vi "get_all_sensor_thicknesses.vi"(8 "error in (no error)":errorcluster, 11 "VISA resource name":refnum<visa-resource-name>) -> (0 "error out":errorcluster, 2 "Thickness array (kA)":dbl[](array[numeric]), 3 "VISA resource name out":refnum<visa-resource-name>)   [LabVIEW 2018]
doc: "Query all sendor thicknesses. Returns thicknesses in kA."
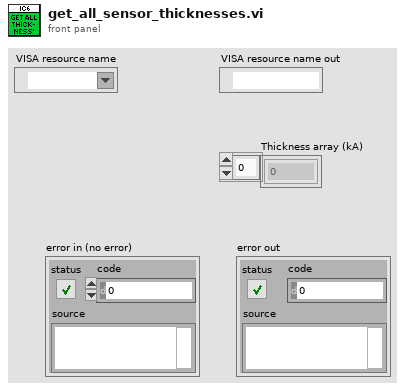
[diagram p1: front panel]
types:
  T1 = enum16{"Source", "General", "Input name", "Process name", "Logic", "Material", "Material name", "Output name", "Process", "Sensor", "Output type", "User message", "Layer", ""}
  T2 = enum16{"Hello", "Query", "Remote action", "Status", "Update"}
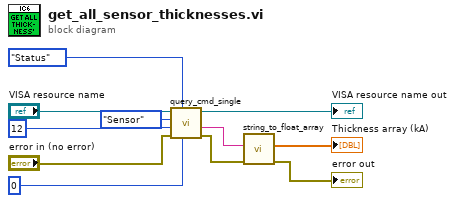
[diagram p0: block diagram]
diagram:
  n1 = call "query_cmd_single.vi"("Parameter"=u8 0 ("Command ID"), "Command group"=T2."Status", "error in (no error)"="error in (no error)", "Command ID"=u8 12, "Command subgroup"=T1."Sensor", "VISA resource name"="VISA resource name") -> ("error out"=w4:errorcluster, "formatted response"=w2:string, "VISA resource name out"=→"VISA resource name out":refnum<visa-resource-name>)  [unwired: 1 in, 2 out]
  n2 = call "string_to_float_array.vi"("error in (no error)"=w4, "Floats"=w2) -> ("error out"=→"error out":errorcluster, "Float array"=→"Thickness array (kA)":sgl[])  [unwired: 8 in]
